vi "BuildTree.vi"() -> ()   [LabVIEW 2016]
panel:
  in  "Tree":dbl[][](array[numeric])=[[1.0, -4074.855712890625, -2495.422607421875, 0.0], [2.0, -3995.446082952127, -2485.7215418602573, 1.0], [3.0, -3928.4179106542683, -2442.0497647220577, 2.0], [4.0, -3859.0751474924227, -2402.1551385541115, 3.0], [5.0, -3802.4779219057964, -2345.615293702038, 4.0], [6.0, -3742.069263739231, -2293.167281170436, 5.0], [7.0, -3672.77094468922, -2253.1955039164422, 6.0], [8.0, -3603.6657385749218, -2212.8907834993447, 7.0], [9.0, -3534.580113450913, -2172.5525088557147, 8.0], [10.0, -3496.5203922124124, -2102.1859143719144, 9.0], [11.0, -3421.5914591897026, -2130.2154522931555, 10.0], [12.0, -3346.003894186188, -2104.013925298733, 11.0], [13.0, -3277.517302162765, -2062.666776509279, 12.0], [14.0, -3208.983825629606, -2021.3973859845944, 13.0], [15.0, -3519.61107162261, -2025.5907413883936, 10.0], [16.0, -3140.245093975219, -1980.470783749054, 14.0], [17.0, -3071.772171708189, -1939.1010011026185, 16.0], [18.0, -3022.1394014153, -2001.843236582822, 17.0], [19.0, -2944.1694400674987, -1983.9355531083372, 18.0], [20.0, -2875.9385159450226, -1942.1678503537817, 19.0], [21.0, -3533.8724989407187, -1946.8721813732973, 15.0], [22.0, -2796.7112680204204, -1931.0753670297627, 20.0], [23.0, -3589.548699320516, -1889.4251561129006, 21.0], [24.0, -2738.8693317675443, -1875.8095510987712, 22.0], [25.0, -2659.3813281882867, -1866.7731089347355, 24.0], [26.0, -2617.893458101461, -1798.3716715546725, 25.0], [27.0, -2553.7234026740616, -1750.5992528756433, 26.0], [28.0, -2480.1819887139936, -1719.1086124764083, 27.0], [29.0, -3584.9971713102927, -1809.5547386057149, 23.0], [30.0, -2605.040856209544, -1689.2272807496508, 27.0], [31.0, -2434.609983161505, -1653.3576253361077, 28.0], [32.0, -2791.7205782939104, -1815.7533629029717, 24.0], [33.0, -3457.9565155004325, -1974.6131413136814, 15.0], [34.0, -2421.9694508872344, -1574.3625815433284, 31.0], [35.0, -2374.8296164751505, -1509.7263996356592, 34.0], [36.0, -2308.5128566051217, -1464.9817087736033, 35.0], [37.0, -3601.8465299701475, -1731.3492457503432, 29.0], [38.0, -2229.248851136565, -1475.8084089671336, 36.0], [39.0, -2151.68903610079, -1495.4164453710252, 38.0], [40.0, -2087.453811461072, -1447.7316897830497, 39.0], [41.0, -2023.2185868213537, -1400.046934195074, 40.0], [42.0, -2417.063062075153, -1441.7827754112213, 35.0], [43.0, -1958.9833621816356, -1352.3621786070985, 41.0], [44.0, -3719.6496319427356, -2188.3696704749273, 7.0], [45.0, -1886.5020524303434, -1386.2215899536834, 43.0], [46.0, -3255.866890350512, -1956.5747183260096, 14.0], [47.0, -1823.8026538786646, -1336.5347162217033, 45.0], [48.0, -1759.4436205382783, -1289.0171949533221, 47.0], [49.0, -1694.7836369960899, -1241.9100136714421, 48.0], [50.0, -1632.2334394039913, -1192.035443185177, 49.0], [51.0, -1595.1057872210595, -1121.1726359913941, 50.0], [52.0, -1528.7872608468076, -1076.4305634025247, 51.0], [53.0, -1569.7150043968538, -1007.692511292346, 52.0], [54.0, -1501.8719340072869, -965.2977262343195, 53.0], [55.0, -1426.4813498710791, -938.5346953222312, 54.0], [56.0, -4074.855712890625, -2495.422607421875, 1.0], [57.0, -3457.9565155004325, -1974.6131413136814, 15.0], [58.0, -1353.6354889703744, -905.4668778914545, 55.0], [59.0, -1289.4629936531828, -857.6977367565644, 58.0], [60.0, -1210.4288331059622, -845.3041308811073, 59.0], [61.0, -1145.519441735295, -798.5412084757492, 60.0], [62.0, -3332.235656727068, -1932.7459222564844, 46.0], [63.0, -1078.6459620045268, -754.6329210040367, 61.0], [64.0, -1008.5426937612098, -793.1755179794031, 63.0], [65.0, -2656.3583097450264, -1627.8553086236584, 30.0], [66.0, -3662.4888087375916, -2284.9849109922975, 6.0], [67.0, -930.9883351395379, -773.5459112899887, 64.0], [68.0, -873.6954562960591, -717.7111010563498, 67.0], [69.0, -816.4025774525803, -661.8762908227109, 68.0], [70.0, -3581.261862592472, -2107.584714548962, 9.0], [71.0, -748.4028323146939, -619.733264576575, 69.0], [72.0, -2081.406416843497, -1345.1454183934663, 41.0], [73.0, -2656.3583097450264, -1627.8553086236584, 30.0], [74.0, -2677.71609658009, -1722.6684146581083, 30.0], [75.0, -3650.7130167180976, -2148.187200759912, 8.0], [76.0, -689.0069451591556, -566.1410208373308, 71.0], [77.0, -615.2520214367194, -597.1282960756863, 76.0], [78.0, -3614.268564152668, -1652.319548377974, 37.0], [79.0, -3120.2753627586953, -1875.4815036358978, 17.0], [80.0, -535.4462494166589, -591.5570527420904, 77.0], [81.0, -3870.993440194968, -2323.047905641713, 4.0], [82.0, -3046.210770145632, -1845.2418587791713, 79.0], [83.0, -2534.972060241506, -1650.62205012491, 30.0], [84.0, -466.23391679698415, -551.436571521852, 80.0], [85.0, -2605.0408562095445, -1689.2272807496502, 83.0], [86.0, -1203.1375656554223, -854.0403237472997, 61.0], [87.0, -2040.1027679111362, -1276.632583210033, 72.0], [88.0, -2279.182890257245, -1390.552191282003, 36.0], [89.0, -1923.68640904426, -1280.5699429599345, 43.0], [90.0, -461.02152261867417, -471.60655870129733, 84.0], [91.0, -484.9521901722836, -395.2696531415445, 90.0], [92.0, -432.1128508449745, -335.20298834772154, 91.0], [93.0, -1256.7998817568207, -780.1142095203654, 60.0], [94.0, -3168.7785538092007, -1811.8620061691765, 79.0], [95.0, -3581.261862592472, -2107.584714548962, 9.0], [96.0, -2435.4681011105718, -1495.5096396695594, 34.0], [97.0, -710.2623540331347, -489.0163970547801, 76.0], [98.0, -369.76061025376737, -285.08115584674226, 92.0], [99.0, -319.19669571606914, -223.08687750894444, 98.0], [100.0, -268.6327811783709, -161.09259917114662, 99.0], [101.0, -3168.7785538092007, -1811.8620061691765, 79.0], [102.0, -1009.9191274091929, -713.68634353405, 63.0], [103.0, -1622.5732089360333, -947.6424470717786, 53.0], [104.0, -393.9897371367454, -585.7990293096639, 84.0], [105.0, -498.2008879816779, -290.12115888819636, 92.0], [106.0, -553.494575721654, -232.30586596224103, 105.0], [107.0, -579.2615039868272, -156.56904923630898, 106.0], [108.0, -218.06886664067267, -99.09832083334881, 100.0], [109.0, -3168.7785538092007, -1811.8620061691765, 79.0], [110.0, -1867.029486372691, -1224.0899189391548, 89.0], [111.0, -1577.706450354954, -1250.5743829197347, 50.0], [112.0, -2435.4681011105718, -1495.5096396695594, 34.0], [113.0, -1686.182766903889, -1132.9637066074465, 50.0], [114.0, -167.5049521029744, -37.104042495550985, 108.0], [115.0, -3674.2638081368355, -1599.3991298301182, 78.0], [116.0, -1674.881473143118, -887.1127395254686, 103.0], [117.0, -2003.5463042167548, -1285.3025049551043, 89.0], [118.0, -1923.68640904426, -1280.5699429599345, 117.0], [119.0, -1512.1443930012608, -1296.4177754158297, 111.0], [120.0, -2435.4681011105718, -1495.5096396695594, 34.0], [121.0, -95.40053864825491, -2.449265619182796, 114.0]]
  in  "k":i32=1
  out "KD-Tree":dbl[][](array[numeric])
  in  "Algorithm":enum16{"RRT", "A*"}(ring)
  in  "Novo nó":dbl[](array[numeric])
  # "x"
  # "y"
  # "F"
  # "right"
  # "left"
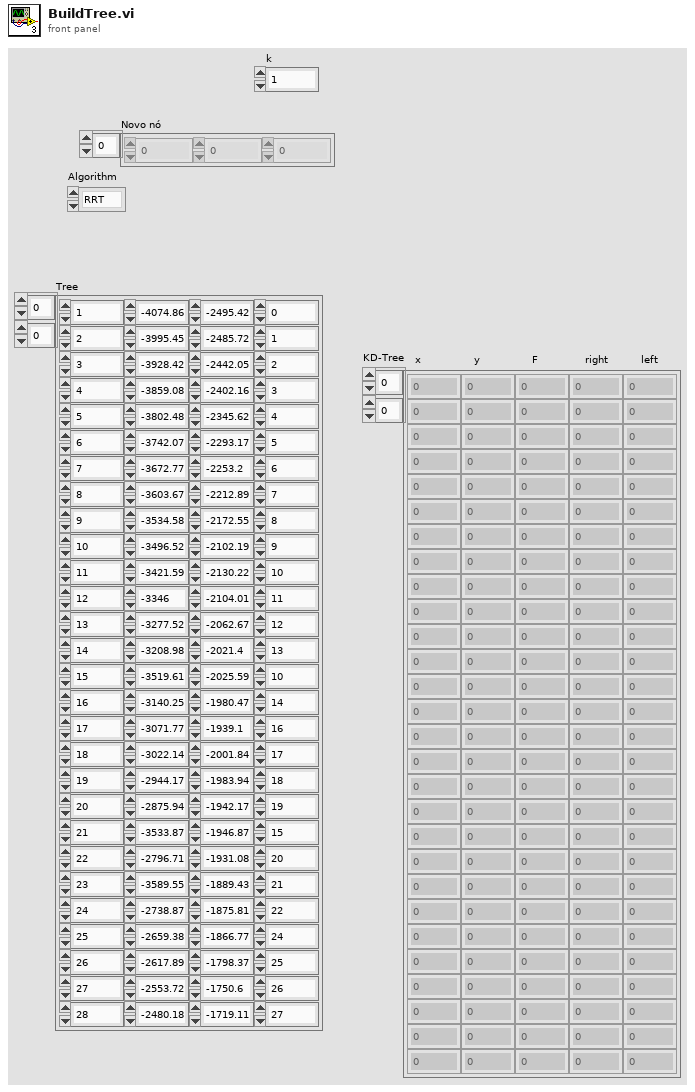
[diagram p1: front panel]
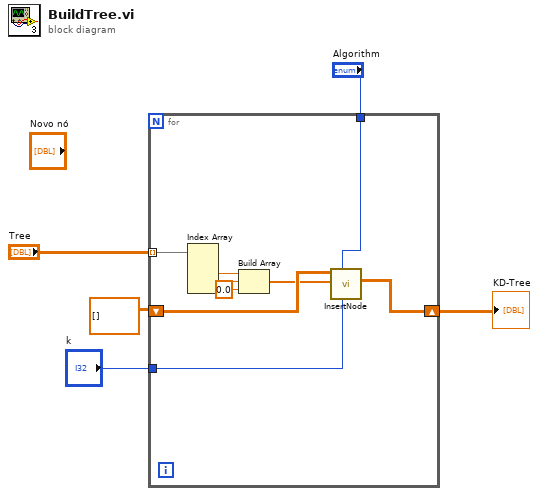
[diagram p0: block diagram]
diagram:
  n1 = for {
    tunnel: "Tree" -> [w14] mode=indexing
    tunnel: "Algorithm" -> [w13]
    tunnel: "k" -> [w12]
    shift-right: [w11] -> w1
    shift-left: dbl[][] [] ("New Tree") -> [w10]
    n2 = Index Array(array=w14) -> (element #2=w9:dbl, element #3=w8:dbl)  [unwired: 4 in, 2 out]
    n3 = Build Array(w9, w8, 0.0 ("element")) -> (w7:dbl[])
    n4 = call "InsertNode.vi"("k"=w12, "Algorithm"=w13, "New Node"=w7, "Tree"=w10) -> ("New Tree"=w11:dbl[][])  [unwired: 7 in]
  }
  "KD-Tree" <- w1
